vi "Do.vi"(8 "error in (no error)":errorcluster, 10 "Actor in":refnum<class "Actor.lvclass">, 11 "Request Check-out Details Msg":refnum<class "Request Check-out Details Msg.lvclass">) -> (0 "error out":errorcluster, 2 "Actor out":refnum<class "Actor.lvclass">)   [LabVIEW 2023, in "Incoming Hotel Management Tool Model Interface.lvlib" / "Request Check-out Details Msg.lvclass"]
doc: "This VI delivers the message to the actor by calling the appropriate method(s) on the actor."
uses:
  Request Check-out Details Msg.lvclass
  Request Check-out Details Msg.lvclass/Request Check-out Details Msg.ctl
  9ef47adc-f318-494c-9b8b-6df3216d6863.vi
  Hotel Management Tool Model/Incoming Hotel Management Tool Model Interface.lvclass
  <vilib>/ActorFramework/Actor/Actor.lvclass
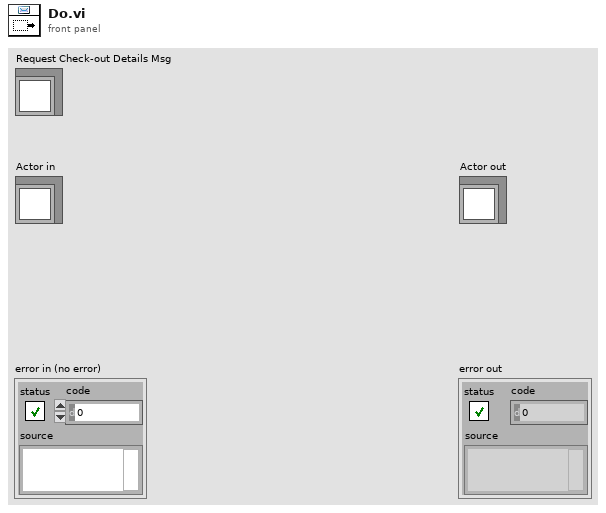
[diagram p1: front panel]
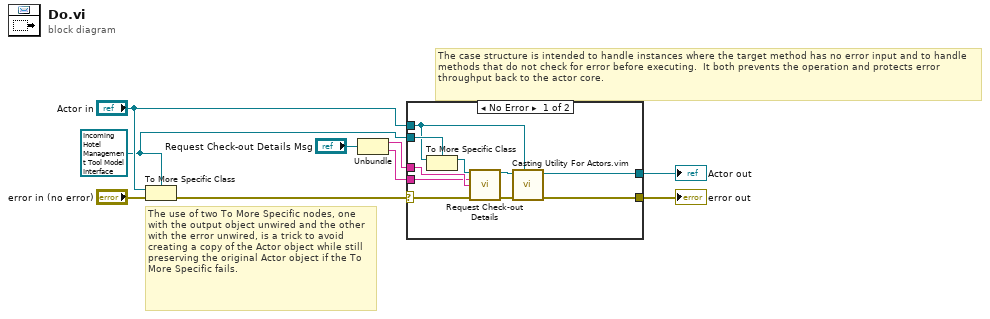
[diagram p0: block diagram]
diagram:
  w3 = refnum<class "Incoming Hotel Management Tool Model Interface.lvclass"> refnum ("Actor in")
  # "The use of two To More Specific nodes, one with the output object unwired and the other with the error unwired, is a trick to avoid creating a copy of the Actor object while still preserving the original Actor object if the To More Specific fails."
  # "The case structure is intended to handle instances where the target method has no error input and to handle methods that do not check for error before executing.  It both prevents the operation and protects error throughput back to the actor core."
  n1 = To More Specific Class(target class=w3, reference="Actor in", error in="error in (no error)") -> (error out=w7:errorcluster)  [unwired: 1 out]
  n2 = Unbundle("Request Check-out Details Msg") -> (w2:string, w1:string)
  n3 = case shown="No Error" w7 {
    selector: w7 -> [w19 w21]
    tunnel: [w13 w21] -> w6
    tunnel: [w14 w20] -> w5
    tunnel: "Actor in" -> [w16 w20]
    tunnel: w3 -> [w17 _]
    tunnel: w2 -> [w11 _]
    tunnel: w1 -> [w10 _]
    frame No Error {
      n4 = To More Specific Class(target class=w17, reference=w16) -> (specific class reference=w18:refnum<class "Incoming Hotel Management Tool Model Interface.lvclass">)  [unwired: 1 in, 1 out]
      n5 = call-dynamic "Request Check-out Details.vi"("Incoming Hotel Management Tool Model Interface in"=w18, "Rooms Manager GUID"=w10, "Room No"=w11, "error in (no error)"=w19) -> ("Incoming Hotel Management Tool Model Interface out"=w15:refnum<class "Incoming Hotel Management Tool Model Interface.lvclass">, "error out"=w12:errorcluster)  [unwired: 10 in]
      n6 = call "Casting Utility For Actors.vim"("type"=w16, "error in (no error)"=w12, "Actor in"=w15) -> ("error out"=w13:errorcluster, "Actor out"=w14:refnum<class "Actor.lvclass">)  [unwired: 7 in]
    }
    frame Error {
      # "If type check fails, pass the original object out again."
    }
  }
  "error out" <- w6
  "Actor out" <- w5
